vi "Throttle to Torque Percent.vi"(10 "Zero Torque Percent":dbl, 11 "Throttle Percent":dbl) -> (1 "Regen Percent":dbl, 2 "Regen?":bool, 3 "Torque Percent":dbl)   [LabVIEW 2015]
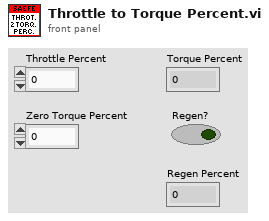
[diagram p1: front panel]
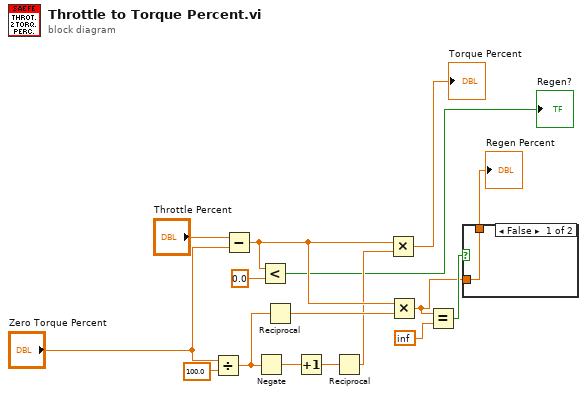
[diagram p0: block diagram]
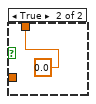
[diagram p2: hidden frame]
diagram:
  n1 = Divide(x="Zero Torque Percent", y=100.0) -> (x/y=w11:dbl)
  n2 = Subtract(x="Throttle Percent", y="Zero Torque Percent") -> (x-y=w16:dbl)
  n3 = Negate(x=w11) -> (-x=w10:dbl)
  n4 = Less?(x=w16, y=0.0) -> (x < y?=→"Regen?":bool)
  n5 = Reciprocal(x=w11) -> (1/x=w15:dbl)
  n6 = Increment(x=w10) -> (x+1=w12:dbl)
  n7 = Reciprocal(x=w12) -> (1/x=w13:dbl)
  n8 = Multiply(x=w16, y=w13) -> (x*y=→"Torque Percent":dbl)
  n9 = Multiply(x=w16, y=w15) -> (x*y=w1:dbl)
  n10 = Equal?(x=w1, y=inf) -> (x = y?=w3:bool)
  n11 = case shown="False" w3 {
    tunnel: [w17 0.0] -> w2
    tunnel: w1 -> [w17 _]
    frame False {
    }
    frame True {
    }
  }
  "Regen Percent" <- w2
